vi "Info Insert Row to 2D Reals Array.vi"(5 "format string (%_20f)":string="%_20f", 6 "source info data":string, 7 "key description":string, 8 "sections in":string[](array[string]), 9 "row index to insert":i32, 10 "row to insert":ext[](array[numeric]), 11 "info data in":string) -> (0 "sections out":string[](array[string]), 3 "info data out":string)   [LabVIEW 2018]
doc: "Addition to infolib: Gets 2D array of reals (if exits in the 'info data in'), inserts one row of reals into it in selected row, writes it back."
uses:
  infolib.lvlibp/Private/Get matrix polymorph parts/Get 2D EXT.vi
  infolib.lvlibp/Private/Add matrix polymorph parts/2D EXT.vi
  infolib.lvlibp
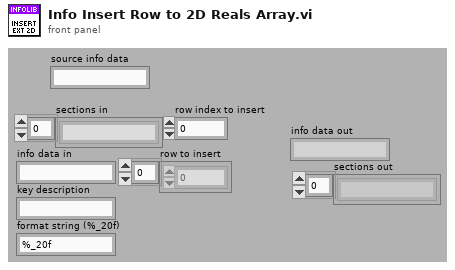
[diagram p1: front panel]
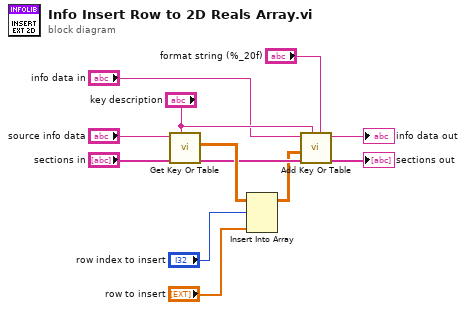
[diagram p0: block diagram]
diagram:
  n1 = call-poly "Get Key Or Table.vi"("key description"="key description", "sections"="sections in", "info data"="source info data") -> ("sections out"=w10:string[], "value"=w12:ext[][])  [unwired: 5 in, 2 out]
  n2 = Insert Into Array(array=w12, index (row)="row index to insert", new element="row to insert") -> (w7:ext[][])  [unwired: 1 in]
  n3 = call-poly "Add Key Or Table.vi"("format string (%_20f)"="format string (%_20f)", "key description"="key description", "sections"=w10, "numeric"=w7, "info data"="info data in") -> ("sections out"=→"sections out":string[], "info data out"=→"info data out":string)  [unwired: 5 in]
